vi "ADS Set Device.vi"(8 "error in (no error)":errorcluster, 10 "CPU:0/Gpu:1":i32, 11 "ref in":u64) -> (0 "error out":errorcluster, 2 "ref out":u64, 3 "dev num":u64)   [LabVIEW 2024]
uses:
  TransformCV-LabVIEW/Test/dependencies_dll_release/TCV_Lib.dll
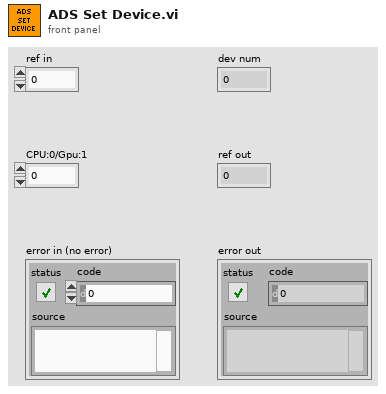
[diagram p1: front panel]
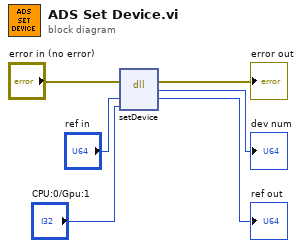
[diagram p0: block diagram]
diagram:
  n1 = dll-call lib="D:/TransformCV-LabVIEW/Test/dependencies_dll_release/TCV_Lib.dll" fn="setDevice"(error in="error in (no error)", "ref"="ref in", "device"="CPU:0/Gpu:1") -> (error out=→"error out":errorcluster, "dev num"=→"dev num":u64, "ref"=→"ref out":u64)  [unwired: 3 in, 1 out]
